vi "TestingRemoteEvents.vi"() -> ()   [LabVIEW 2020]
panel:
  out "text":string
  in  "String":string
  in  "stop":bool
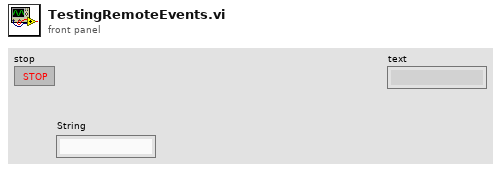
[diagram p1: front panel]
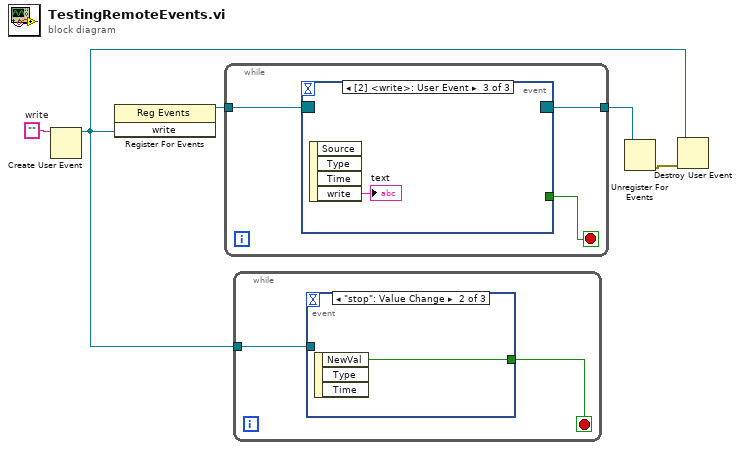
[diagram p0: block diagram]
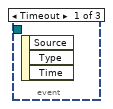
[diagram p2: hidden frame]
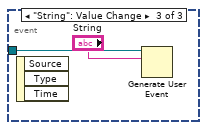
[diagram p3: hidden frame]
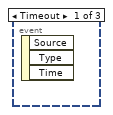
[diagram p4: hidden frame]
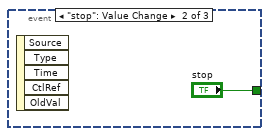
[diagram p5: hidden frame]
diagram:
  w5 = ""  # write
  n1 = Create User Event(user event datatype=w5) -> (user event=w1:refnum<user-event>)  [unwired: 1 in, 1 out]
  n2 = register-events(w1) -> (reference out=w4:refnum<event-registration>)  [unwired: 2 in, 1 out]
  n3 = while {
    tunnel: w4 -> [w8]
    tunnel: [w7] -> w3
    stop <- w6 stop-if-true
    n4 = event shown="[2] <write>: User Event" {
      selector: w8 -> [_ _ _]
      dyn-events: [_ _ _] -> w7
      timeout: _ -> [_ _ _]
      tunnel: [_ "stop" _] -> w6
      event Timeout {
        n5 = event-data() -> ()  [unwired: 1 in, 3 out]
      }
      event "stop": Value Change {
        n6 = event-data() -> ()  [unwired: 1 in, 5 out]
      }
      event User Event {
        n7 = event-data() -> ("write"=→"text":string)  [unwired: 1 in, 3 out]
      }
    }
  }
  n8 = while {
    tunnel: w1 -> [w12]
    stop <- w11 stop-if-true
    n9 = event shown="[1] \"stop\": Value Change" {
      selector: _ -> [_ _ _]
      dyn-events: _ -> [_ _ _]
      timeout: _ -> [_ _ _]
      tunnel: w12 -> [_ _ w15]
      tunnel: [_ w13 _] -> w11
      event Timeout {
        n10 = event-data() -> ()  [unwired: 1 in, 3 out]
      }
      event "stop": Value Change {
        n11 = event-data() -> ("NewVal"=w13:bool)  [unwired: 1 in, 2 out]
      }
      event "String": Value Change {
        n12 = event-data() -> ()  [unwired: 1 in, 3 out]
        n13 = Generate User Event(user event=w15, event data cluster="String") -> ()  [unwired: 2 in, 2 out]
      }
    }
  }
  n14 = Unregister For Events(event registration refnum=w3) -> (error out=w2:errorcluster)  [unwired: 1 in]
  n15 = Destroy User Event(user event=w1, error in=w2) -> ()  [unwired: 1 out]
